vi "BuildMenu.vi"(8 "error in (no error)":errorcluster, 11 "Waveform_Task in":refnum<class "Waveform_Task.lvclass">) -> (0 "error out":errorcluster, 3 "Waveform_Task out":refnum<class "Waveform_Task.lvclass">)   [LabVIEW 2025, in "Waveform_Task.lvlib" / "Waveform_Task.lvclass"]
uses:
  Waveform_Task.lvclass
  Waveform_Task.lvclass/Waveform_Task.ctl
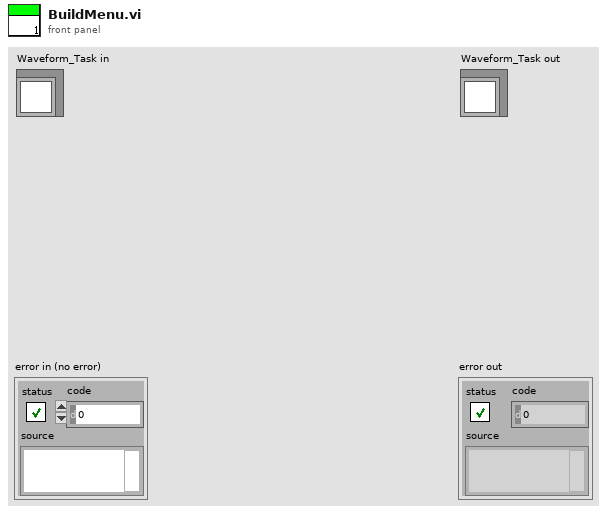
[diagram p1: front panel]
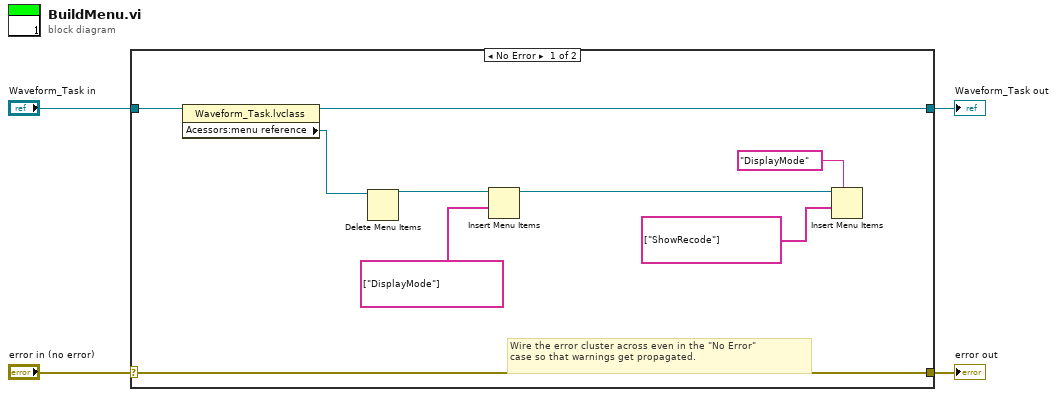
[diagram p0: block diagram]
diagram:
  n1 = case shown="No Error" "error in (no error)" {
    selector: "error in (no error)" -> [w12 w15]
    tunnel: [w12 w15] -> w3
    tunnel: [w6 w14] -> w1
    tunnel: "Waveform_Task in" -> [w13 w14]
    frame No Error {
      # "Wire the error cluster across even in the \"No Error\"\ncase so that warnings get propagated."
      n2 = property class="Waveform_Task.lvclass"(reference=w13) -> (reference out=w6:refnum<class "Waveform_Task.lvclass">, "Acessors:menu reference"=w5:refnum<k9>)  [unwired: 1 in, 1 out]
      n3 = Delete Menu Items(9:w5) -> (3:w10:refnum<k9>)  [unwired: 3 in, 1 out]
      n4 = Insert Menu Items(7:string[] ["DisplayMode"] ("item tags"), 9:w10) -> (3:w9:refnum<k9>)  [unwired: 4 in, 2 out]
      n5 = Insert Menu Items(5:"DisplayMode" ("menu tag"), 7:string[] ["ShowRecode"] ("item tags"), 9:w9) -> ()  [unwired: 3 in, 3 out]
    }
    frame Error {
    }
  }
  "error out" <- w3
  "Waveform_Task out" <- w1
